vi "whilelooping arrays.vi"() -> ()   [LabVIEW 2018]
panel:
  out "Waveform Chart 2":dbl[](graph)
  out "Waveform Chart":dbl[](graph)
  out "Array 2":dbl[](array[numeric])
  out "Array":dbl[](array[numeric])
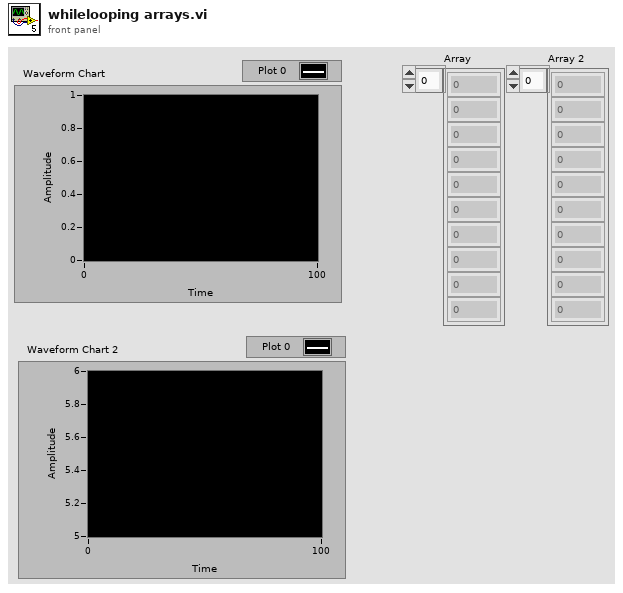
[diagram p1: front panel]
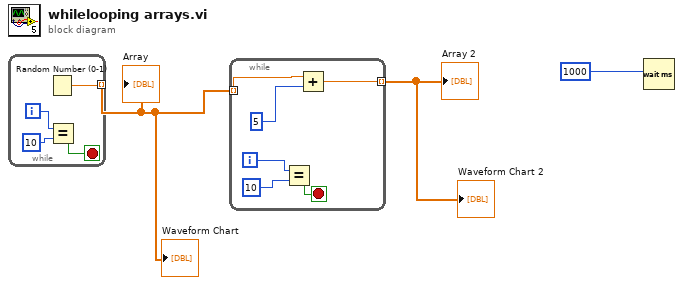
[diagram p0: block diagram]
diagram:
  n1 = while {
    tunnel: [w7] -> w3 mode=indexing
    i -> [w6]
    stop <- w4 stop-if-true
    n2 = Random Number (0-1)() -> (number: 0 to 1=w7:dbl)
    n3 = Equal?(x=w6, y=10) -> (x = y?=w4:bool)
  }
  "Array" <- w3
  "Waveform Chart" <- w3
  n4 = while {
    tunnel: w3 -> [w9] mode=indexing
    tunnel: [w8] -> w2 mode=indexing
    i -> [w12]
    stop <- w11 stop-if-true
    n5 = Equal?(x=w12, y=10) -> (x = y?=w11:bool)
    n6 = Add(x=w9, y=5) -> (x+y=w8:dbl)
  }
  "Array 2" <- w2
  "Waveform Chart 2" <- w2
  n7 = Wait (ms)(milliseconds to wait=1000) -> ()  [unwired: 1 out]
